vi "zPos.vi"(11 "DistanceIn":dbl) -> (3 "DistanceOut":dbl)   [LabVIEW 2012]
uses:
  2013NewCan/Robot Global Data.vi
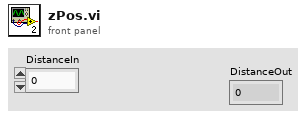
[diagram p1: front panel]
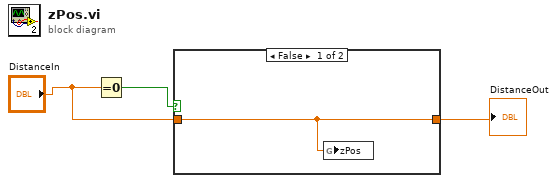
[diagram p0: block diagram]
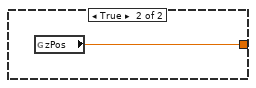
[diagram p2: hidden frame]
diagram:
  n1 = Equal To 0?(x="DistanceIn") -> (x = 0?=w3:bool)
  n2 = case shown="False" w3 {
    tunnel: [w4 w5] -> w2
    tunnel: "DistanceIn" -> [w4 _]
    frame False {
      n3 = global write "Robot Global Data.vi" "zPos"(w4) -> ()
    }
    frame True {
      n4 = global read "Robot Global Data.vi" "zPos"() -> (w5:dbl)
    }
  }
  "DistanceOut" <- w2
